vi "Zoom_1.vi"(2 "Fator Zoom":i32(slide), 4 "IMAGEM Cam1":T1) -> (1 "Image Dst Out 2":T1)   [LabVIEW 2012]
uses:
  <vilib>/vision/Image Controls.llb/IMAQ Image.ctl
  <vilib>/vision/NI_Vision_Development_Module.lvlib
panel:
  out "error out":errorcluster
  out "appended array":i32[](array[numeric])
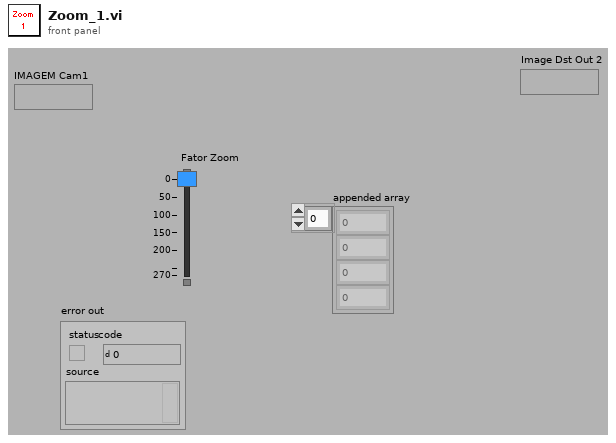
[diagram p1: front panel]
types:
  T1 = typedef "IMAQ Image.ctl" = refnum<image>
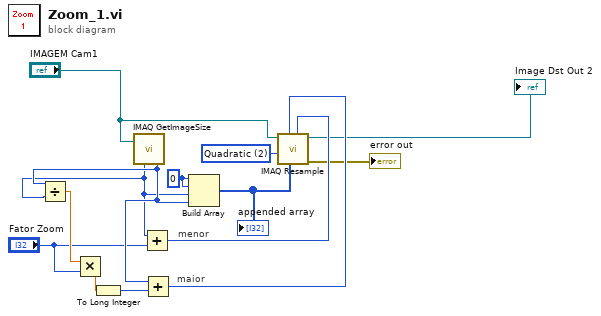
[diagram p0: block diagram]
diagram:
  w3 = u32 2 items=["Zero Order", "Bi-Linear", "Quadratic", "Cubic Spline"] ("Interpolation Type")
  w13 = 0 ("element")
  # "menor"
  # "maior"
  n1 = call "IMAQ GetImageSize"("Image"="IMAGEM Cam1") -> ("Y Resolution"=w9:i32, "X Resolution"=w8:i32)  [unwired: 3 in, 1 out]
  n2 = Divide(x=w9, y=w8) -> (x/y=w7:dbl)
  n3 = Multiply(x=w7, y="Fator Zoom") -> (x*y=w5:dbl)
  n4 = To Long Integer(number=w5) -> (32bit integer=w4:i32)
  n5 = Add(x=w8, y="Fator Zoom") -> (x+y=w11:i32)
  n6 = Add(x=w9, y=w4) -> (x+y=w10:i32)
  n7 = Build Array(w13, w13, w8, w9) -> (w14:i32[])
  "appended array" <- w14
  n8 = call "IMAQ Resample"("X Resolution"=w11, "Optional Rectangle"=w14, "Y Resolution"=w10, "Interpolation Type"=w3, "Image Src"="IMAGEM Cam1") -> ("error out"=→"error out":errorcluster, "Image Dst Out"=→"Image Dst Out 2":T1)  [unwired: 5 in]
